vi "Configure Power Measurement List Single Retrigger.vi"(7 "Retrigger (Off)":bool, 8 "error in (no error)":errorcluster, 9 "Index (0)":i32, 10 "Instance (1)":i32=1, 11 "VISA resource name":refnum<visa-resource-name>) -> (0 "error out":errorcluster, 3 "VISA resource name out":refnum<visa-resource-name>)   [LabVIEW 2015, in "Rohde&Schwarz CMXP GPRF.lvlib"]
doc: "Enables the retrigger mechanism after a selected frequency/level step.\n\nAttribute:\nRSCMXPGPRF_ATTR_POWER_MEASUREMENT_LIST_SINGLE_RETRIGGER\n\nRemote-control command:\nCONFigure:GPRF:MEAS<i>:POWer:LIST:RETRigger"
uses:
  <instrlib>/Rohde&Schwarz CMXP GPRF/Rohde&Schwarz CMXP GPRF.lvlib
  <instrlib>/Rohde&Schwarz CMXP GPRF/Private/rsidr_core.llb/rsidr_core.lvlib
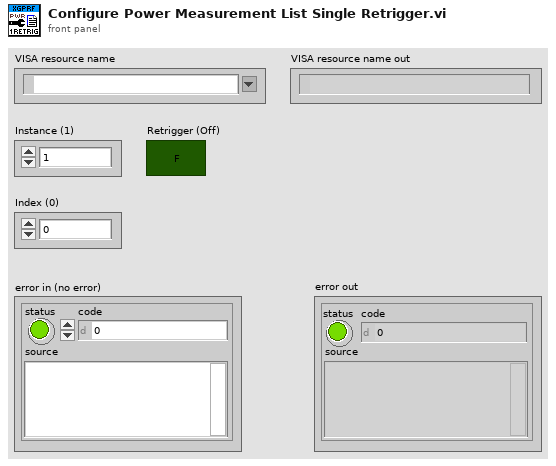
[diagram p1: front panel]
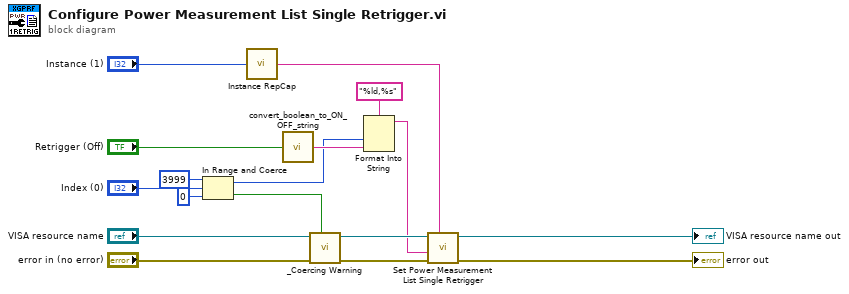
[diagram p0: block diagram]
diagram:
  n1 = In Range and Coerce(upper limit=3999, x="Index (0)", lower limit=0) -> (coerced(x)=w2:i32, In Range?=w3:bool)
  n2 = call <instrlib>:"Instance RepCap.vi"("instance  in"="Instance (1)") -> ("instance out"=w5:string)
  n3 = call <instrlib>:"convert_boolean_to_ON_OFF_string.vi"("boolean value in"="Retrigger (Off)") -> ("string value out"=w10:string)  [unwired: 4 in]
  n4 = call <instrlib>:"_Coercing Warning.vi"("In Range?"=w3, "error in (no error)"="error in (no error)", "VISA resource name"="VISA resource name") -> ("error out"=w9:errorcluster, "VISA resource name out"=w8:refnum<visa-resource-name>)  [unwired: 7 in]
  n5 = Format Into String(format string="%ld,%s", w2, w10) -> (resulting string=w1:string)  [unwired: 2 in, 1 out]
  n6 = call "Set Power Measurement List Single Retrigger"("Repeated Capabilities"=w5, "error in (no error)"=w9, "Power Measurement List Single Retrigger ()"=w1, "instrument handle"=w8) -> ("error out"=→"error out":errorcluster, "instrument handle out"=→"VISA resource name out":refnum<visa-resource-name>)  [unwired: 6 in]
